vi "Combo box-Edit values.vi"(9 "Index of property key":i32[](array[numeric]), 11 "Combo box ref":refnum<vi>) -> ()   [LabVIEW 2013]
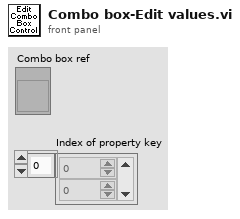
[diagram p1: front panel]
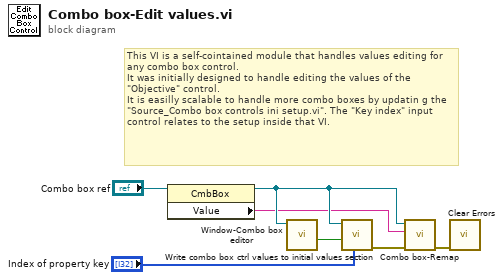
[diagram p0: block diagram]
diagram:
  # "This VI is a self-cointained module that handles values editing for any combo box control.\nIt was initially designed to handle editing the values of the \"Objective\" control.\nIt is easilly scalable to handle more combo boxes by updatin g the \"Source_Combo box controls ini setup.vi\". The \"Key index\" input control relates to the setup inside that VI."
  n1 = property class="CmbBox"(reference="Combo box ref") -> (reference out=w5:refnum<vi>, "Value"=w3:string)  [unwired: 1 in, 1 out]
  n2 = call "Window-Combo box editor.vi"("Combo box ref"=w5) -> ("Cancelled"=w7:bool)  [unwired: 10 in]
  n3 = call "Write combo box ctrl values to initial values section.vi"("Index of property keys"="Index of property key", "Cancelled"=w7, "Combo box ref"=w5) -> ("error out"=w6:errorcluster)  [unwired: 8 in]
  n4 = call "Combo box-Remap.vi"("error in (no error)"=w6, "Value"=w3, "ComboBox in"=w5) -> ("error out"=w4:errorcluster)  [unwired: 8 in]
  n5 = call <vilib>:"Clear Errors.vi"("error in (no error)"=w4) -> ()  [unwired: 6 in, 1 out]
